vi "LookUpTableAlg.vi"(0 "ImageIn":T2, 5 "Function":T1(ring), 7 "Power Value":sgl, 11 "error In":errorcluster) -> (4 "Image Dst Out":T2, 15 "error out":errorcluster)   [LabVIEW 2019]
uses:
  <vilib>/vision/Image Controls.llb/IMAQ Image.ctl
  <vilib>/vision/NI_Vision_Development_Module.lvlib
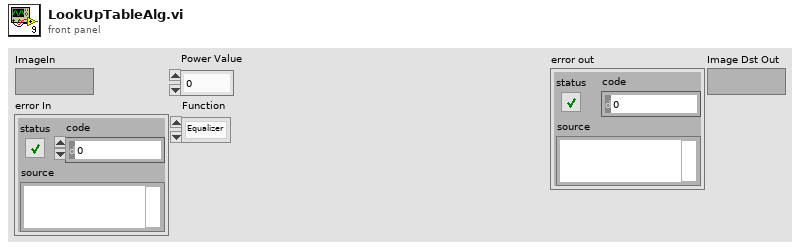
[diagram p1: front panel]
types:
  T1 = enum16{"Equalizer", "Reverse", "Logarithmic", "Exponential", "Square", "Square Root", "Power X", "Power 1/X"}
  T2 = typedef "IMAQ Image.ctl" = refnum<image>
  T3 = enum32{"Linear", "Log", "Exp", "Square", "Square root", "Power X", "Power 1/X"}
  T4 = cluster{"histogram":u32[], "Minimal Value":sgl, "Maximal Value":sgl, "Starting Value":sgl, "Interval Width":sgl, "Mean Value":sgl, "Standard  Variation":sgl, "Area (pixels)":i32}
  T5 = typedef "Image Type" = u32
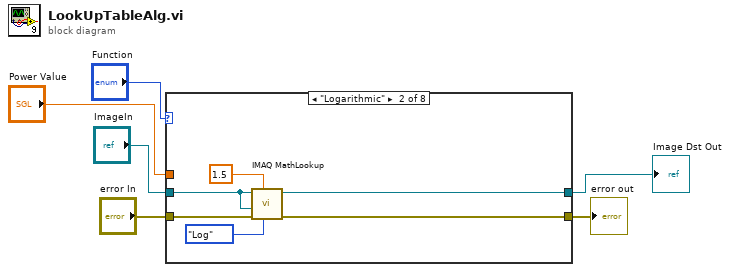
[diagram p0: block diagram]
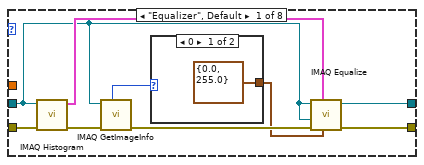
[diagram p2: hidden frame]
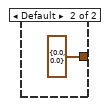
[diagram p3: hidden frame]
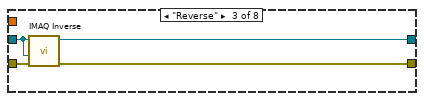
[diagram p4: hidden frame]
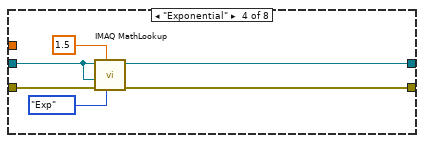
[diagram p5: hidden frame]
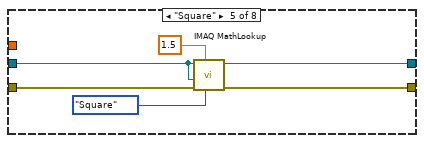
[diagram p6: hidden frame]
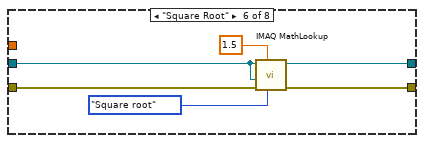
[diagram p7: hidden frame]
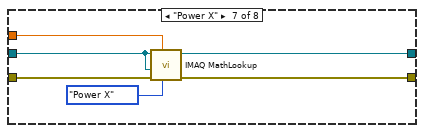
[diagram p8: hidden frame]
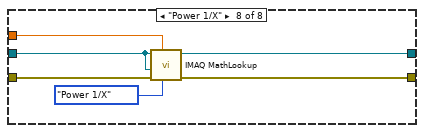
[diagram p9: hidden frame]
diagram:
  n1 = case shown="\"Logarithmic\"" "Function" {
    tunnel: "ImageIn" -> [w10 w21 w27 w31 w37 w43 w49 w56]
    tunnel: "error In" -> [w9 w20 w26 w30 w36 w42 w48 w54]
    tunnel: [w8 w19 w24 w28 w34 w40 w47 w53] -> w4
    tunnel: [w7 w18 w25 w29 w35 w41 w46 w52] -> w3
    tunnel: "Power Value" -> [_ _ _ _ _ _ w50 w55]
    frame "Equalizer", Default {
      n2 = call "IMAQ Histogram"("error in (no error)"=w9, "Image"=w10) -> ("error out"=w13:errorcluster, "Histogram Report"=w15:T4)  [unwired: 3 in, 5 out]
      n3 = call "IMAQ GetImageInfo"("error in (no error)"=w13, "Image"=w10) -> ("error out"=w12:errorcluster, "Image Type"=w14:T5)  [unwired: 8 out]
      n4 = case shown="0" w14 {
        tunnel: [cluster{"Minimum":sgl, "Maximum":sgl} {"Minimum"=0.0, "Maximum"=255.0} ("Range") cluster{"Minimum":sgl, "Maximum":sgl} {"Minimum"=0.0, "Maximum"=0.0} ("Range")] -> w11
        frame 0 {
        }
        frame Default {
        }
      }
      n5 = call "IMAQ Equalize"("Range"=w11, "Histogram Report"=w15, "error in (no error)"=w12, "Image Dst"=w10, "Image Src"=w10) -> ("error out"=w8:errorcluster, "Image Dst Out"=w7:T2)  [unwired: 1 in, 4 out]
    }
    frame "Logarithmic" {
      n6 = call "IMAQ MathLookup"("Operator"=T3."Log" ("Operator (Lookup Table 1)"), "X Value"=sgl 1.5 ("X Value (Lookup Table 1)"), "error in (no error)"=w20, "Image Dst"=w21, "Image Src"=w21) -> ("error out"=w19:errorcluster, "Image Dst Out"=w18:T2)  [unwired: 2 in, 3 out]
    }
    frame "Reverse" {
      n7 = call "IMAQ Inverse"("error in (no error)"=w26, "Image Dst"=w27, "Image Src"=w27) -> ("error out"=w24:errorcluster, "Image Dst Out"=w25:T2)  [unwired: 1 in, 6 out]
    }
    frame "Exponential" {
      n8 = call "IMAQ MathLookup"("Operator"=T3."Exp" ("Operator (Lookup Table 1)"), "X Value"=sgl 1.5 ("X Value (Lookup Table 1)"), "error in (no error)"=w30, "Image Dst"=w31, "Image Src"=w31) -> ("error out"=w28:errorcluster, "Image Dst Out"=w29:T2)  [unwired: 2 in, 3 out]
    }
    frame "Square" {
      n9 = call "IMAQ MathLookup"("Operator"=T3."Square" ("Operator (Lookup Table 1)"), "X Value"=sgl 1.5 ("X Value (Lookup Table 1)"), "error in (no error)"=w36, "Image Dst"=w37, "Image Src"=w37) -> ("error out"=w34:errorcluster, "Image Dst Out"=w35:T2)  [unwired: 2 in, 3 out]
    }
    frame "Square Root" {
      n10 = call "IMAQ MathLookup"("Operator"=T3."Square root" ("Operator (Lookup Table 1)"), "X Value"=sgl 1.5 ("X Value (Lookup Table 1)"), "error in (no error)"=w42, "Image Dst"=w43, "Image Src"=w43) -> ("error out"=w40:errorcluster, "Image Dst Out"=w41:T2)  [unwired: 2 in, 3 out]
    }
    frame "Power X" {
      n11 = call "IMAQ MathLookup"("Operator"=T3."Power X" ("Operator (Lookup Table 1)"), "X Value"=w50, "error in (no error)"=w48, "Image Dst"=w49, "Image Src"=w49) -> ("error out"=w47:errorcluster, "Image Dst Out"=w46:T2)  [unwired: 2 in, 3 out]
    }
    frame "Power 1/X" {
      n12 = call "IMAQ MathLookup"("Operator"=T3."Power 1/X" ("Operator (Lookup Table 1)"), "X Value"=w55, "error in (no error)"=w54, "Image Dst"=w56, "Image Src"=w56) -> ("error out"=w53:errorcluster, "Image Dst Out"=w52:T2)  [unwired: 2 in, 3 out]
    }
  }
  "error out" <- w4
  "Image Dst Out" <- w3
